vi "Error Handler.vi"(8 "error in (no error)":errorcluster, 11 "QControlWizard in":refnum<class "QControl Creation Wizard.lvclass">) -> (0 "error out":errorcluster, 3 "QControlWizard out":refnum<class "QControl Creation Wizard.lvclass">)   [LabVIEW 2015, in "QControl Creation Wizard.lvclass"]
doc: "<b> </b> <b> </b>\n©2016 Q Software Innovations, LLC (QSI)\nwritten by Quentin Alldredge\nproduced in LabVIEW 2015\n\nsupport@qsoftwareinnovations.com\nwww.qsoftwareinnovations.com\n\nAll rights reserved.\n\nRedistribution and use in source and binary forms, with or without modification, are permitted provided that the following conditions are met:\n\n * Redistributions of source code must retain the above copyright notice, this list of conditions and the following disclaimer.\n * Redistributions in binary form must reproduce the above copyright notice, this list of conditions and the following disclaimer in the documentation and/or other materials provided with the distribution.\n * Neither the name of Q Software Innovations, LLC. nor the names of its contributors may be used to endorse or promote products derived from this software without specific prior written permission.\n\nTHIS SOFTWARE IS PROVIDED BY THE COPYRIGHT HOLDERS AND CONTRIBUTORS \"AS IS\" AND ANY EXPRESS OR IMPLIED WARRANTIES, INCLUDING, BUT NOT LIMITED TO, THE IMPLIED WARRANTIES OF MERCHANTABILITY AND FITNESS FOR A PARTICULAR PURPOSE ARE DISCLAIMED. IN NO EVENT SHALL THE COPYRIGHT OWNER OR CONTRIBUTORS BE LIABLE FOR ANY DIRECT, INDIRECT, INCIDENTAL, SPECIAL, EXEMPLARY, OR CONSEQUENTIAL DAMAGES (INCLUDING, BUT NOT LIMITED TO, PROCUREMENT OF SUBSTITUTE GOODS OR SERVICES; LOSS OF USE, DATA, OR PROFITS; OR BUSINESS INTERRUPTION) HOWEVER CAUSED AND ON ANY THEORY OF LIABILITY, WHETHER IN CONTRACT, STRICT LIABILITY, OR TORT (INCLUDING NEGLIGENCE OR OTHERWISE) ARISING IN ANY WAY OUT OF THE USE OF THIS SOFTWARE, EVEN IF ADVISED OF THE POSSIBILITY OF SUCH DAMAGE."
uses:
  QControl Creation Wizard.lvclass
  Error Message Type.ctl
  Warning Dialog/Warning Dialog.lvclass
  Error Dialog/Error Dialog.lvclass
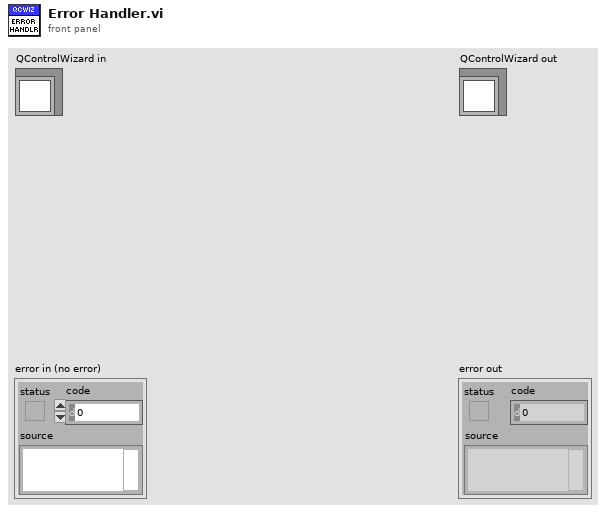
[diagram p1: front panel]
types:
  T1 = typedef "QControl Creation Wizard.lvclass/Error Message Type.ctl" = enum16{"Warning", "Error"}
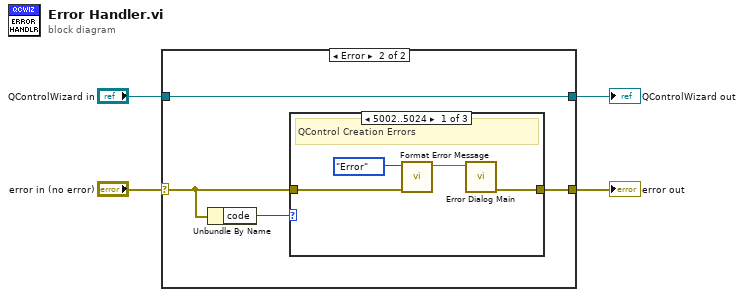
[diagram p0: block diagram]
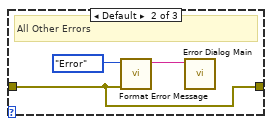
[diagram p3: hidden frame]
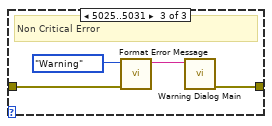
[diagram p4: hidden frame]
diagram:
  n1 = case shown="Error" "error in (no error)" {
    selector: "error in (no error)" -> [w5 w8]
    tunnel: [w5 w7] -> w3
    tunnel: [w6 w10] -> w1
    tunnel: "QControlWizard in" -> [w6 w10]
    frame No Error {
    }
    frame Error {
      n2 = Unbundle By Name(w8) -> ("code"=w9:i32)
      n3 = case shown="5002..5024" w9 {
        tunnel: w8 -> [w14 w15 w21]
        tunnel: [w11 w15 w18] -> w7
        frame 5002..5024 {
          # "QControl Creation Errors"
          n4 = call "Format Error Message.vi"("error in (no error)"=w14, "Message Type"=Error_Message_Type."Error") -> ("message"=w13:string)  [unwired: 9 in]
          n5 = call "Error Dialog Main.vi"("Message in"=w13) -> ("error out"=w11:errorcluster)  [unwired: 10 in]
        }
        frame Default {
          # "All Other Errors"
          n6 = call "Format Error Message.vi"("error in (no error)"=w15, "Message Type"=Error_Message_Type."Error") -> ("message"=w17:string)  [unwired: 9 in]
          n7 = call "Error Dialog Main.vi"("Message in"=w17) -> ()  [unwired: 10 in, 1 out]
        }
        frame 5025..5031 {
          # "Non Critical Error"
          n8 = call "Format Error Message.vi"("error in (no error)"=w21, "Message Type"=Error_Message_Type."Warning") -> ("message"=w20:string)  [unwired: 9 in]
          n9 = call "Warning Dialog Main.vi"("Message in"=w20) -> ("error out"=w18:errorcluster)  [unwired: 10 in]
        }
      }
    }
  }
  "error out" <- w3
  "QControlWizard out" <- w1
